vi "File_MoveFilesAndFolders.vi"(1 "Source":path, 3 "TargetDirectory":path, 5 "error in (no error)":errorcluster, 6 "Remove original?":bool=TRUE, 8 "Ignore errors?":bool, 10 "Include source folder?":bool) -> (19 "error out":errorcluster)   [LabVIEW 2020]
doc: "Moves files and folders to the specified directory and then delete them."
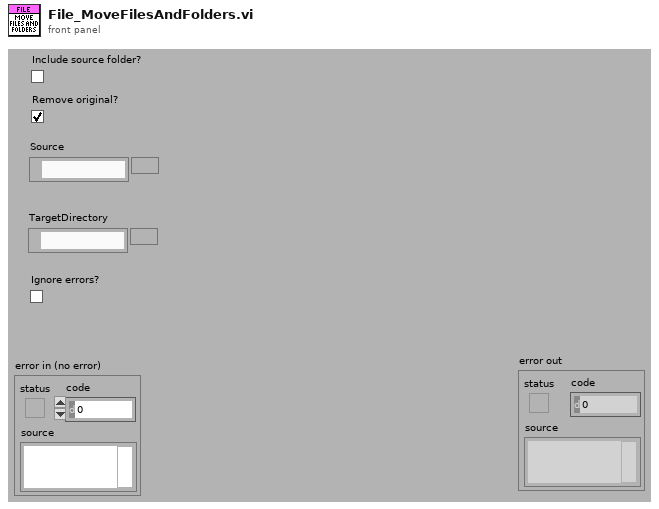
[diagram p1: front panel]
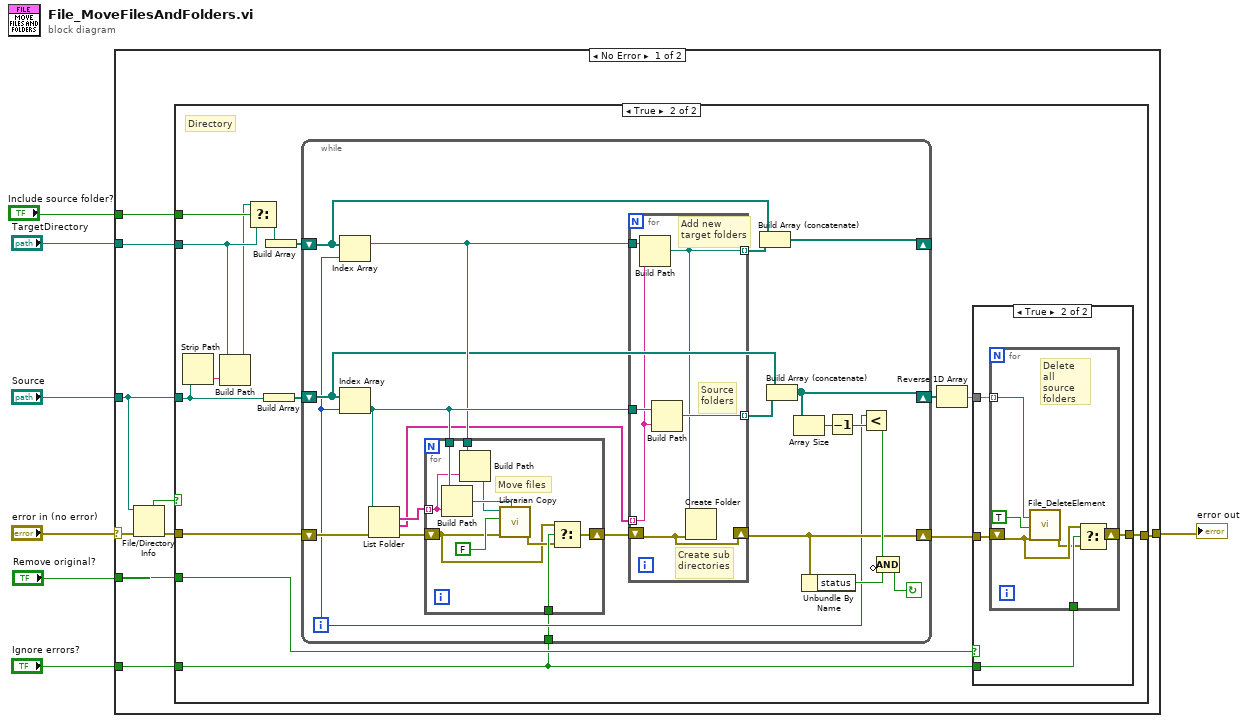
[diagram p0: block diagram]
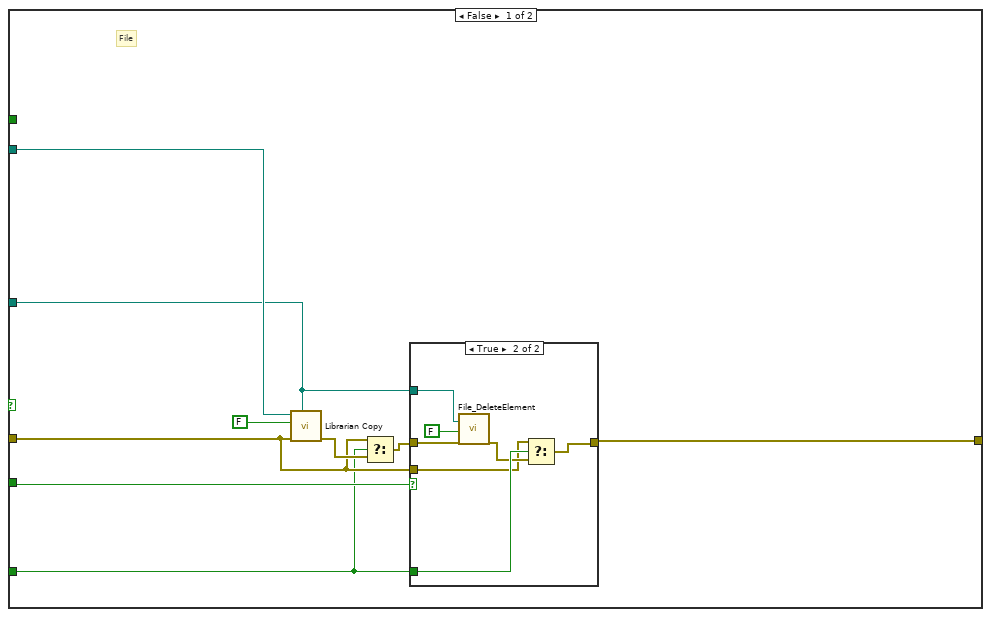
[diagram p2: hidden frame]
diagram:
  n1 = case shown="No Error" "error in (no error)" {
    selector: "error in (no error)" -> [w16 w97]
    tunnel: [w10 w97] -> w6
    tunnel: "Source" -> [w13 _]
    tunnel: "TargetDirectory" -> [w12 _]
    tunnel: "Remove original?" -> [w11 _]
    tunnel: "Ignore errors?" -> [w9 _]
    tunnel: "Include source folder?" -> [w8 _]
    frame No Error {
      n2 = File/Directory Info(path=w13, error in=w16) -> (directory=w14:bool, error out=w15:errorcluster)  [unwired: 5 out]
      n3 = case shown="True" w14 {
        tunnel: w13 -> [w21 w39]
        tunnel: w12 -> [w25 w35]
        tunnel: [w17 w42] -> w10
        tunnel: w11 -> [w20 w41]
        tunnel: w15 -> [w19 w47]
        tunnel: w9 -> [w18 w40]
        tunnel: w8 -> [_ w38]
        frame False {
          # "File"
          n4 = call <vilib>:"Librarian Copy.vi"("source"=w21, "error in (no error)"=w19, "remove original (F)"=FALSE, "destination"=w25) -> ("error out"=w24:errorcluster)  [unwired: 2 in, 5 out]
          n5 = Select(t=w19, s=w18, f=w24) -> (s? t:f=w22:errorcluster)
          n6 = case shown="True" w20 {
            tunnel: w22 -> [w26 w33]
            tunnel: w21 -> [_ w32]
            tunnel: w19 -> [_ w28]
            tunnel: w18 -> [_ w30]
            tunnel: [w26 w27] -> w17
            frame False {
            }
            frame True {
              n7 = call <resource>:"File_DeleteElement.vi"("Filepath"=w32, "Recursive?"=FALSE, "error in (no error)"=w33) -> ("error out"=w29:errorcluster)  [unwired: 2 in, 14 out]
              n8 = Select(t=w28, s=w30, f=w29) -> (s? t:f=w27:errorcluster)
            }
          }
        }
        frame True {
          # "Directory"
          n9 = Strip Path(path=w39) -> (name=w36:string)  [unwired: 1 out]
          n10 = Build Path(base path=w35, name or relative path=w36) -> (appended path=w34:path)
          n11 = Select(t=w34, s=w38, f=w35) -> (s? t:f=w37:path)
          n12 = Build Array(w39) -> (w46:path[])
          n13 = Build Array(w37) -> (w45:path[])
          n14 = while {
            tunnel: w40 -> [w49]
            shift-left: w45 -> [w55]
            shift-right: [w68] -> _
            shift-left: w46 -> [w54]
            shift-right: [w66] -> w48
            shift-left: w47 -> [w62]
            shift-right: [w53] -> w43
            i -> [w50]
            stop <- w63 continue-if-true
            n15 = Index Array(array=w55, index=w50) -> (element=w58:path)
            n16 = Index Array(array=w54, index=w50) -> (element=w60:path)
            n17 = List Folder(path=w60, error in=w62) -> (filenames=w59:string[], folder names=w56:string[], error out=w61:errorcluster)  [unwired: 3 out]
            n18 = for {
              shift-right: [w77] -> w57
              shift-left: w61 -> [w76]
              tunnel: w59 -> [w83] mode=indexing
              tunnel: w58 -> [w85]
              tunnel: w60 -> [w84]
              tunnel: w49 -> [w79]
              # "Move files"
              n19 = Build Path(base path=w84, name or relative path=w83) -> (appended path=w82:path)
              n20 = Build Path(base path=w85, name or relative path=w83) -> (appended path=w81:path)
              n21 = call <vilib>:"Librarian Copy.vi"("source"=w82, "error in (no error)"=w76, "remove original (F)"=FALSE, "destination"=w81) -> ("error out"=w78:errorcluster)  [unwired: 2 in, 5 out]
              n22 = Select(t=w76, s=w79, f=w78) -> (s? t:f=w77:errorcluster)
            }
            n23 = for {
              tunnel: [w71] -> w69 mode=indexing
              tunnel: [w75] -> w67 mode=indexing
              tunnel: w60 -> [w74]
              tunnel: w58 -> [w73]
              shift-right: [w70] -> w53
              shift-left: w57 -> [w70]
              tunnel: w56 -> [w72] mode=indexing
              # "Source\nfolders"
              # "Add new\ntarget folders"
              # "Create sub\ndirectories"
              n24 = Build Path(base path=w73, name or relative path=w72) -> (appended path=w71:path)
              n25 = Build Path(base path=w74, name or relative path=w72) -> (appended path=w75:path)
              n26 = Create Folder(path (use dialog)=w71, error in=w70) -> ()  [unwired: 4 out]
            }
            n27 = Build Array (concatenate)(w55, w69) -> (w68:path[])
            n28 = Build Array (concatenate)(w54, w67) -> (w66:path[])
            n29 = Array Size(array=w66) -> (size(s)=w52:i32)
            n30 = Unbundle By Name(w53) -> ("status"=w64:bool)
            n31 = Decrement(x=w52) -> (x-1=w51:i32)
            n32 = Less?(x=w50, y=w51) -> (x < y?=w65:bool)
            n33 = Compound Arithmetic op=AND(w65, invert w64) -> (w63:bool)
          }
          n34 = Reverse 1D Array(array=w48) -> (reversed array=w44:path[])
          n35 = case shown="True" w41 {
            tunnel: w43 -> [w86 w90]
            tunnel: w44 -> [_ w89]
            tunnel: [w86 w88] -> w42
            tunnel: w40 -> [_ w87]
            frame False {
            }
            frame True {
              n36 = for {
                shift-right: [w92] -> w88
                shift-left: w90 -> [w94]
                tunnel: w89 -> [w96] mode=indexing
                tunnel: w87 -> [w95]
                # "Delete all\nsource\nfolders"
                n37 = call <resource>:"File_DeleteElement.vi"("Filepath"=w96, "Recursive?"=TRUE, "error in (no error)"=w94) -> ("error out"=w93:errorcluster)  [unwired: 2 in, 14 out]
                n38 = Select(t=w94, s=w95, f=w93) -> (s? t:f=w92:errorcluster)
              }
            }
          }
        }
      }
    }
    frame Error {
    }
  }
  "error out" <- w6
